vi "Lambda ctrl age.vi"(8 "CO/HC Eq O2":dbl, 9 "Flow rate":dbl, 10 "Lambda_t":dbl, 11 "O2Eq Measured":dbl) -> (2 "Air MFC":dbl)   [LabVIEW 2011]
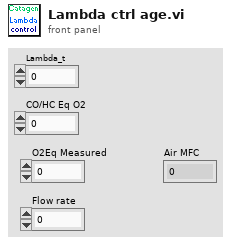
[diagram p1: front panel]
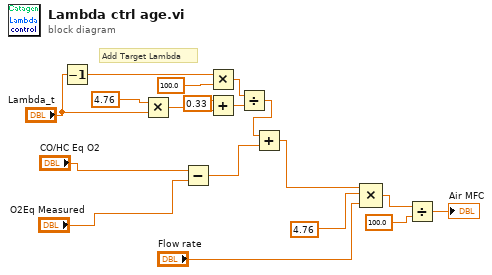
[diagram p0: block diagram]
diagram:
  # "Add Target Lambda"
  n1 = Decrement(x="Lambda_t") -> (x-1=w13:dbl)
  n2 = Multiply(x=4.76, y="Lambda_t") -> (x*y=w10:dbl)
  n3 = Subtract(x="CO/HC Eq O2", y="O2Eq Measured") -> (x-y=w4:dbl)
  n4 = Multiply(x=w13, y=100.0) -> (x*y=w11:dbl)
  n5 = Add(x=0.33, y=w10) -> (x+y=w9:dbl)
  n6 = Divide(x=w11, y=w9) -> (x/y=w5:dbl)
  n7 = Add(x=w5, y=w4) -> (x+y=w3:dbl)
  n8 = Compound Arithmetic op=MULTIPLY(w3, 4.76 ("y"), "Flow rate") -> (w17:dbl)
  n9 = Divide(x=w17, y=100.0) -> (x/y=→"Air MFC":dbl)
